vi "SaveFileSettingControl.vi"(8 "error in":errorcluster, 10 "This VI":refnum<vi>, 11 "Path to was selected by user":path caption="selected path") -> (0 "error out":errorcluster)   [LabVIEW 2013]
uses:
  <vilib>/regexp/Match Regular Expression.xnode
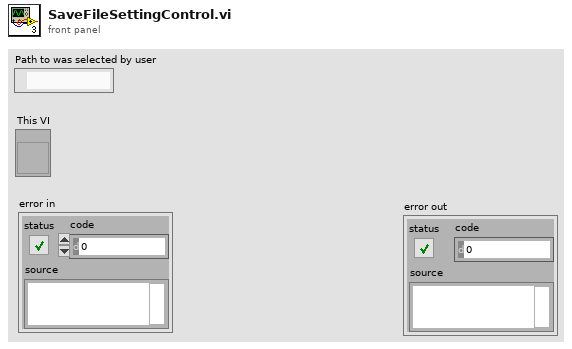
[diagram p1: front panel]
types:
  T1 = enum16{"open", "replace", "create", "open or create", "replace or create", "replace or create with confirmation"}
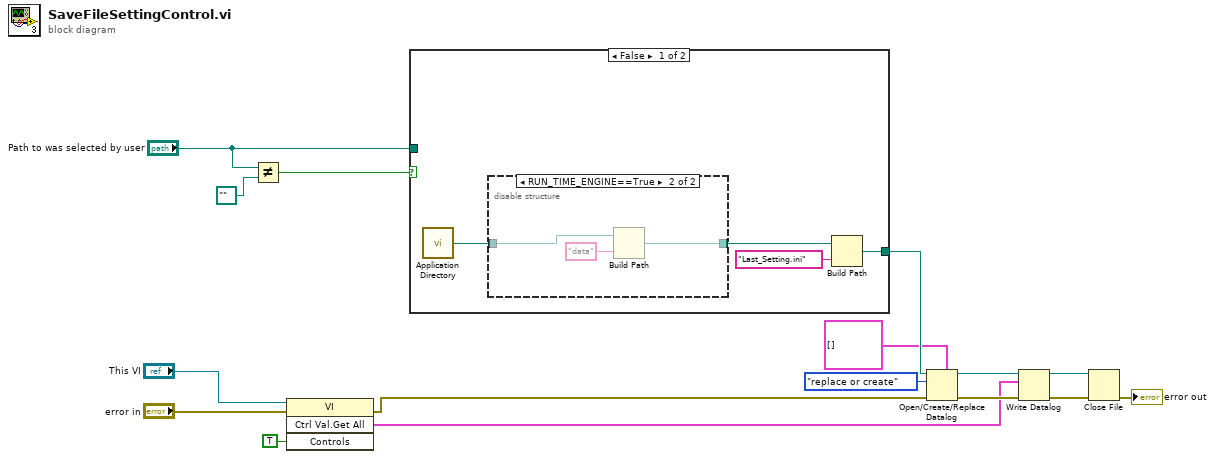
[diagram p0: block diagram]
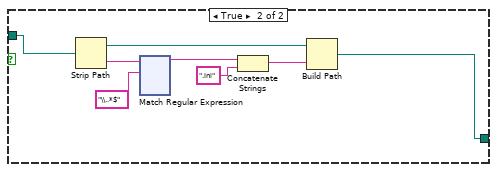
[diagram p3: hidden frame]
diagram:
  n1 = Not Equal?(x="Path to was selected by user", y=path "" ("Path to folder was selected by user")) -> (x != y?=w1:bool)
  n2 = invoke class="VI" method="Ctrl Val.Get All"(reference="This VI", error in="error in", "Controls"=TRUE) -> (error out=w4:errorcluster, "Get All Control Values Variant"=w7:cluster{"Name":string, "Variant Data":variant}[])  [unwired: 1 in, 2 out]
  n3 = case shown="False" w1 {
    tunnel: [w19 w25] -> w14
    tunnel: "Path to was selected by user" -> [_ w30]
    frame False {
      n4 = call <vilib>:"Application Directory.vi"() -> ("Application Directory"=w18:path)
      n5 = disable-structure shown="RUN_TIME_ENGINE==True" {
        disable-tunnel: w18 -> [w21 w24]
        disable-tunnel: [w21 w22] -> w17
        frame condition #0 (active) {
        }
        frame condition #1 {
          n6 = Build Path(base path=w24, name or relative path="data") -> (appended path=w22:path)
        }
      }
      n7 = Build Path(base path=w17, name or relative path="Last_Setting.ini") -> (appended path=w19:path)
    }
    frame True {
      n8 = Strip Path(path=w30) -> (stripped path=w27:path, name=w32:string)
      n9 = xnode "Match Regular Expression"("input string"=w32, "regular expression"="\\..*$") -> ("before match"=w29:string)  [unwired: 4 in, 4 out]
      n10 = Concatenate Strings(w29, ".ini") -> (w26:string)
      n11 = Build Path(base path=w27, name or relative path=w26) -> (appended path=w25:path)
    }
  }
  n12 = Open/Create/Replace Datalog(5:cluster{"Name":string, "Variant Data":variant}[] [] ("Control Value:Get All"), 8:w4, 10:T1."replace or create" ("operation (0:open)"), 11:w14) -> (0:w11:errorcluster, 3:w12:refnum<k1>)  [unwired: 2 in, 1 out]
  n13 = Write Datalog(4:w11, 6:w7, 7:w12) -> (0:w9:errorcluster, 3:w10:refnum<k1>)
  n14 = Close File(refnum=w10, error in=w9) -> (error out=→"error out":errorcluster)  [unwired: 1 out]
